vi "RT_DynamicPressure_v2.vi"(9 "i":i32, 10 "V_wind [m/s]":dbl[][](array[numeric]), 11 "output cluster 2":T2) -> (3 "output cluster":T1)   [LabVIEW 2017]
uses:
  <vilib>/Analysis/_algsub.llb/Vector Norm Type.ctl
  <vilib>/Analysis/_algsub.llb/Real Vector Norm.vi
  <vilib>/Analysis/NI_AALPro.lvlib
panel:
  out "air flow velocity [m/s]":dbl
  out "Temp [K]":dbl
  out "Pdin":dbl
  out "rho (kg/m^3)":dbl
  out "Patm (Pa)":dbl
  out "p (Pa)":dbl
  out "T(ºC)":dbl
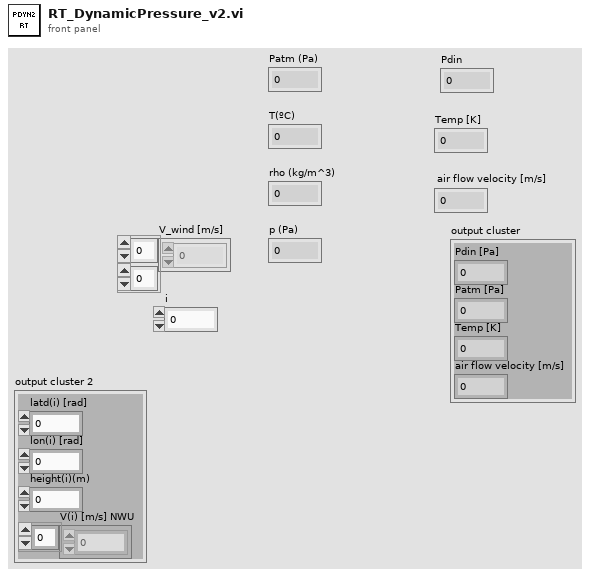
[diagram p1: front panel]
types:
  T1 = cluster{"Pdin [Pa]":dbl, "Patm [Pa]":dbl, "Temp [K]":dbl, "air flow velocity [m/s]":dbl}
  T2 = cluster{"latd(i) [rad]":dbl, "lon(i) [rad]":dbl, "height(i)(m)":dbl, "V(i) [m/s] NWU":dbl[]}
  T3 = typedef "NI_AALPro.lvlib/Vector Norm Type.ctl" = u16
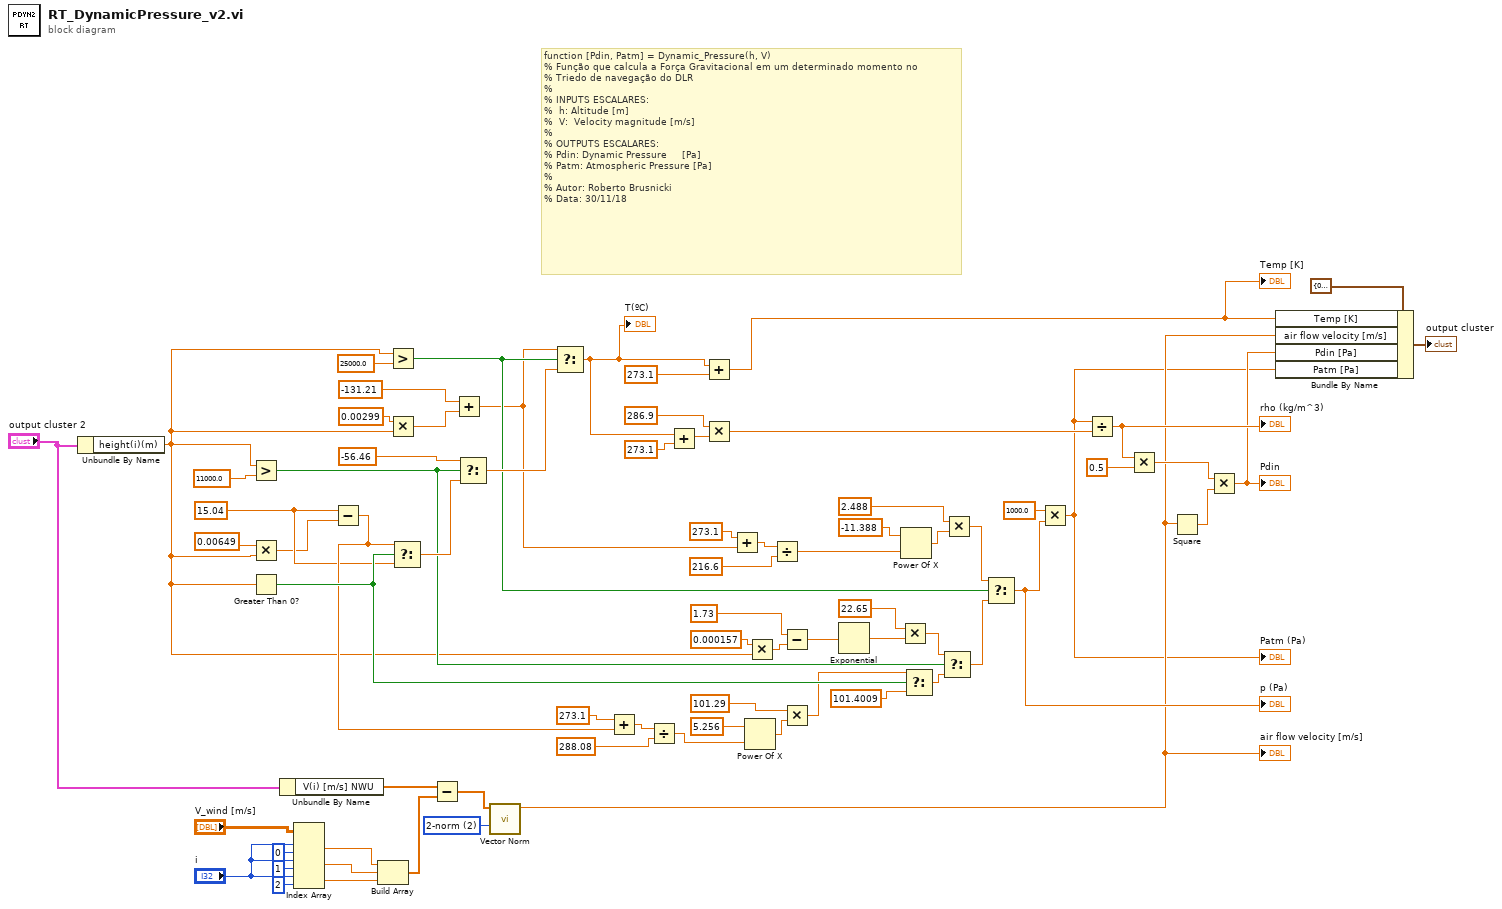
[diagram p0: block diagram]
diagram:
  w27 = T3 2 items=["1-norm"=1, "2-norm"=2, "Inf-norm"=3, "-Inf-norm"=4, "User Defined"=5] ("norm type")
  w54 = 15.04 ("x")
  # "function [Pdin, Patm] = Dynamic_Pressure(h, V)\n% Função que calcula a Força Gravitacional em um determinado momento no \n% Triedo de navegação do DLR\n%\n% INPUTS ESCALARES:\n%  h: Altitude [m]\n%  V:  Velocity magnitude [m/s]\n%\n% OUTPUTS ESCALARES:\n% Pdin: Dynamic Pressure     [Pa]\n% Patm: Atmospheric Pressure [Pa]\n%\n% Autor: Roberto Brusnicki\n% Data: 30/11/18"
  n1 = Unbundle By Name("output cluster 2") -> ("height(i)(m)"=w9:dbl)
  n2 = Greater?(x=w9, y=11000.0) -> (0:w49:bool)
  n3 = Multiply(x=0.00649 ("y"), y=w9) -> (x*y=w51:dbl)
  n4 = Greater Than 0?(x=w9) -> (x > 0?=w63:bool)
  n5 = Unbundle By Name("output cluster 2") -> ("V(i) [m/s] NWU"=w8:dbl[])
  n6 = Index Array(array="V_wind [m/s]", index (row) #1="i", index (col) #1=0 ("disabled index (col)"), index (row) #2="i", index (col) #2=1 ("disabled index (col)"), index (row) #3="i", index (col) #3=2 ("disabled index (col)")) -> (element #1=w12:dbl, element #2=w15:dbl, element #3=w14:dbl)
  n7 = Subtract(x=w54, y=w51) -> (x-y=w61:dbl)
  n8 = Build Array(w12, w15, w14) -> (w13:dbl[])
  n9 = Greater?(x=w9, y=25000.0) -> (0:w32:bool)
  n10 = Multiply(x=0.00299 ("y"), y=w9) -> (x*y=w30:dbl)
  n11 = Select(t=w61, s=w63, f=w54) -> (s? t:f=w53:dbl)
  n12 = Subtract(x=w8, y=w13) -> (x-y=w22:dbl[])
  n13 = Add(x=-131.21 ("y"), y=w30) -> (x+y=w21:dbl)
  n14 = Select(t=-56.46, s=w49, f=w53) -> (s? t:f=w40:dbl)
  n15 = call-poly <vilib>:"Vector Norm.vi"("norm type"=w27, "Input Vector"=w22) -> ("norm"=w5:dbl)  [unwired: 8 in, 1 out]
  "air flow velocity [m/s]" <- w5
  n16 = Select(t=w21, s=w32, f=w40) -> (s? t:f=w10:dbl)
  "T(ºC)" <- w10
  n17 = Add(x=273.1 ("y"), y=w61) -> (x+y=w59:dbl)
  n18 = Divide(x=w59, y=288.08) -> (x/y=w23:dbl)
  n19 = Add(x=w10, y=273.1) -> (x+y=w68:dbl)
  n20 = Add(x=w10, y=273.1) -> (x+y=w3:dbl)
  "Temp [K]" <- w3
  n21 = Multiply(x=286.9, y=w68) -> (x*y=w70:dbl)
  n22 = Add(x=273.1 ("y"), y=w21) -> (x+y=w34:dbl)
  n23 = Power Of X(1:w23, 2:5.256 ("x")) -> (0:w56:dbl)
  n24 = Multiply(x=0.000157 ("y"), y=w9) -> (x*y=w43:dbl)
  n25 = Divide(x=w34, y=216.6) -> (x/y=w25:dbl)
  n26 = Subtract(x=1.73, y=w43) -> (x-y=w45:dbl)
  n27 = Multiply(x=101.29, y=w56) -> (x*y=w62:dbl)
  n28 = Exponential(1:w45) -> (0:w46:dbl)
  n29 = Multiply(x=22.65, y=w46) -> (x*y=w48:dbl)
  n30 = Power Of X(1:w25, 2:-11.388 ("x")) -> (0:w41:dbl)
  n31 = Select(t=w62, s=w63, f=101.4009) -> (s? t:f=w55:dbl)
  n32 = Select(t=w48, s=w49, f=w55) -> (s? t:f=w50:dbl)
  n33 = Multiply(x=2.488, y=w41) -> (x*y=w37:dbl)
  n34 = Select(t=w37, s=w32, f=w50) -> (s? t:f=w65:dbl)
  "p (Pa)" <- w65
  n35 = Multiply(x=1000.0, y=w65) -> (x*y=w4:dbl)
  "Patm (Pa)" <- w4
  n36 = Divide(x=w4, y=w70) -> (x/y=w72:dbl)
  "rho (kg/m^3)" <- w72
  n37 = Multiply(x=w72, y=0.5 ("x")) -> (x*y=w73:dbl)
  n38 = Square(x=w5) -> (x^2=w74:dbl)
  n39 = Multiply(x=w73, y=w74) -> (x*y=w6:dbl)
  "Pdin" <- w6
  n40 = Bundle By Name(cluster=T1 {"Pdin [Pa]"=0.0, "Patm [Pa]"=0.0, "Temp [K]"=0.0, "air flow velocity [m/s]"=0.0} ("output cluster 3"), "Temp [K]"=w3, "air flow velocity [m/s]"=w5, "Pdin [Pa]"=w6, "Patm [Pa]"=w4) -> (→"output cluster":T1)
